vi "Write.vi"(7 "Wait Until Done?":bool, 8 "error in (no error)":errorcluster, 9 "Sample Rate [Hz]":dbl=1000.0 min=1000.0 max=1600000.0, 10 "Values":dbl[][](array[numeric]), 11 "AO (N Samples) Ref In":T1) -> (0 "error out":errorcluster, 3 "AO (N Samples) Ref Out":T1)   [LabVIEW 2021, in "AO Block.lvlib"]
doc: "Writes values to one or more analog output channels. Use this VI to write multiple samples for each channel at one time."
uses:
  <vilib>/myRIO/Instrument Drivers/Onboard IO/AO Block/AO Block.lvlib
  <vilib>/myRIO/Instrument Drivers/Onboard IO/AO Block/typedefs/AO Block Reference.ctl
  <vilib>/myRIO/Common/Instrument Driver Framework/Utilities/typedefs/myRIO Generic Hardware Reference.ctl
  <vilib>/myRIO/Common/Instrument Driver Framework/Utilities/typedefs/Hardware Version Enum.ctl
  <vilib>/myRIO/Common/Instrument Driver Framework/Utilities/typedefs/myRIO v1.0 Reference.ctl
  <vilib>/myRIO/Common/Instrument Driver Framework/Utilities/typedefs/Generic FPGA Reference.ctl
  <vilib>/myRIO/Common/Instrument Driver Framework/myRIO v1.0/AO Block/typedefs/AO Block Channels List.ctl
  <vilib>/myRIO/Common/Instrument Driver Framework/myRIO v1.0/AO Block/typedefs/AO Block Channels Enum.ctl
  <vilib>/myRIO/Common/Instrument Driver Framework/Utilities/typedefs/Analog Scaling Constants.ctl
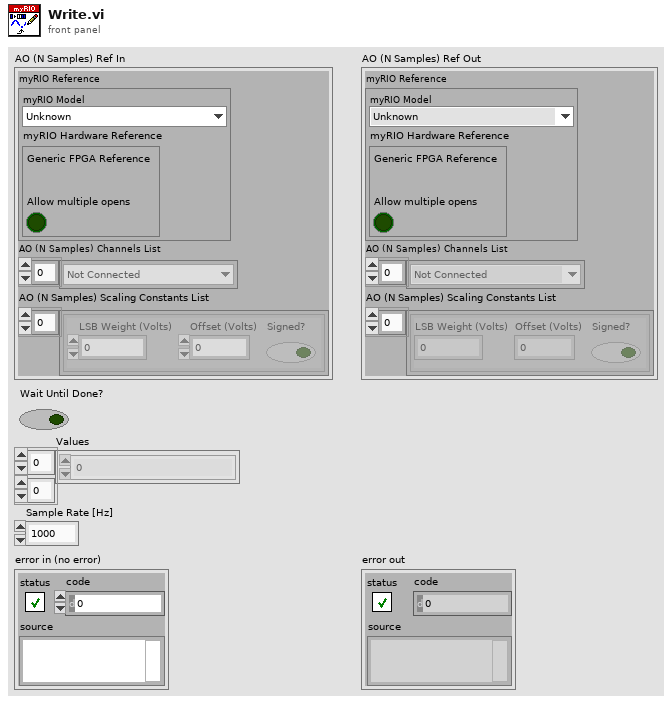
[diagram p1: front panel]
types:
  T1 = typedef "AO Block.lvlib/AO Block Reference.ctl" = cluster{"myRIO Reference":T2, "AO (N Samples) Channels List":T6, "AO (N Samples) Scaling Constants List":T8[]}
  T2 = typedef "myRIO Generic Hardware Reference.ctl" = cluster{"myRIO Model":T3, "myRIO Hardware Reference":T4}
  T3 = typedef "Hardware Version Enum.ctl" = enum16{"Unknown", "myRIO-1900", "myRIO-1950", "roboRIO", "NI ELVIS RIO CM", "ELVIS III"}
  T4 = typedef "myRIO v1.0 Reference.ctl" = cluster{"Generic FPGA Reference":T5, "Allow multiple opens":bool}
  T5 = typedef "Generic FPGA Reference.ctl" = refnum<k20>
  T6 = typedef "AO Block Channels List.ctl" = T7[]
  T7 = typedef "AO Block Channels Enum.ctl" = enum16{"Not Connected", "A/AO0 (N Samples)", "A/AO1 (N Samples)", "B/AO0 (N Samples)", "B/AO1 (N Samples)"}
  T8 = typedef "Analog Scaling Constants.ctl" = cluster{"LSB Weight (Volts)":dbl, "Offset (Volts)":dbl, "Signed?":bool}
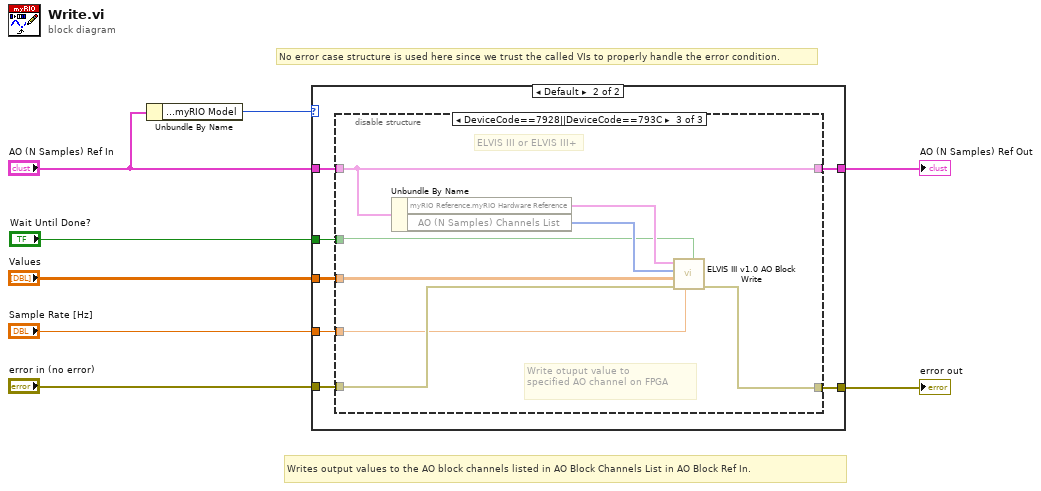
[diagram p0: block diagram]
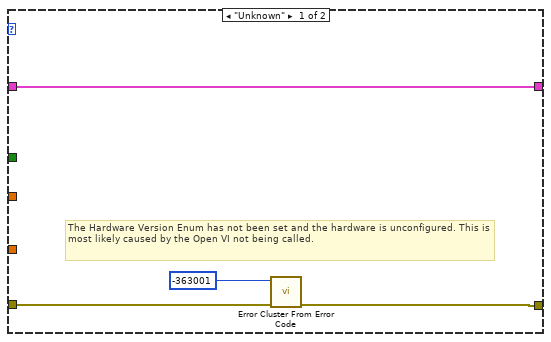
[diagram p2: hidden frame]
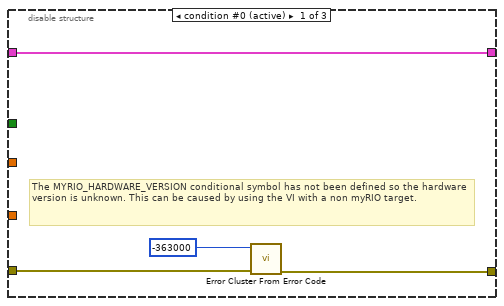
[diagram p3: hidden frame]
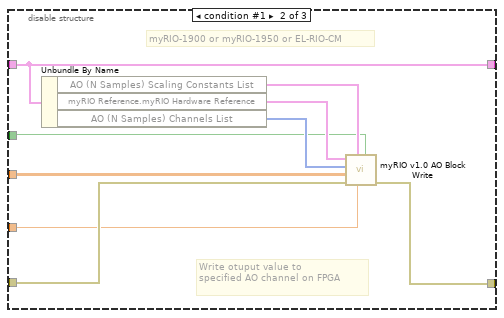
[diagram p4: hidden frame]
diagram:
  # "No error case structure is used here since we trust the called VIs to properly handle the error condition."
  # "Writes output values to the AO block channels listed in AO Block Channels List in AO Block Ref In."
  n1 = Unbundle By Name("AO (N Samples) Ref In") -> ("myRIO Reference.myRIO Model"=w3:T3)
  n2 = case shown="Default" w3 {
    tunnel: [w11 w19] -> w5
    tunnel: "AO (N Samples) Ref In" -> [w9 w18]
    tunnel: "error in (no error)" -> [w10 w17]
    tunnel: [w9 w16] -> w6
    tunnel: "Values" -> [_ w15]
    tunnel: "Sample Rate [Hz]" -> [_ w14]
    tunnel: "Wait Until Done?" -> [_ w13]
    frame "Unknown" {
      # "The Hardware Version Enum has not been set and the hardware is unconfigured. This is most likely caused by the Open VI not being called."
      n3 = call <vilib>:"Error Cluster From Error Code.vi"("error in (no error)"=w10, "error code (0)"=-363001) -> ("error out"=w11:errorcluster)  [unwired: 7 in]
    }
    frame Default {
      n4 = disable-structure shown="DeviceCode==7928||DeviceCode==793C" {
        disable-tunnel: w18 -> [w20 w26 w38]
        disable-tunnel: [w23 w30 w37] -> w19
        disable-tunnel: w17 -> [w21 w32 w36]
        disable-tunnel: [w20 w26 w38] -> w16
        disable-tunnel: w15 -> [_ w29 w34]
        disable-tunnel: w14 -> [_ w27 w35]
        disable-tunnel: w13 -> [_ w24 w33]
        frame condition #0 (active) {
          # "The MYRIO_HARDWARE_VERSION conditional symbol has not been defined so the hardware version is unknown. This can be caused by using the VI with a non myRIO target."
          n5 = call <vilib>:"Error Cluster From Error Code.vi"("error in (no error)"=w21, "error code (0)"=-363000) -> ("error out"=w23:errorcluster)  [unwired: 7 in]
        }
        frame condition #1 {
          # "myRIO-1900 or myRIO-1950 or EL-RIO-CM"
          # "Write otuput value to \nspecified AO channel on FPGA"
          n6 = Unbundle By Name(w26) -> ("AO (N Samples) Scaling Constants List"=w25:T8[], "myRIO Reference.myRIO Hardware Reference"=w28:T4, "AO (N Samples) Channels List"=w31:T6)
          n7 = call <vilib>:"myRIO v1.0 AO Block Write.vi"("Wait Until Done?"=w24, "AO FIFO Sample Rate"=w27, "Scale Constants Array"=w25, "error in (no error)"=w32, "dbl Scaled Value List"=w29, "AO (N Samples) Channel List"=w31, "myRIO Ref In"=w28) -> ("error out"=w30:errorcluster)  [unwired: 3 in, 1 out]
        }
        frame condition #2 {
          # "ELVIS III or ELVIS III+"
          # "Write otuput value to \nspecified AO channel on FPGA"
          n8 = Unbundle By Name(w38) -> ("myRIO Reference.myRIO Hardware Reference"=w39:T4, "AO (N Samples) Channels List"=w40:T6)
          n9 = call <vilib>:"ELVIS III v1.0 AO Block Write.vi"("Wait Until Done?"=w33, "AO FIFO Sample Rate"=w35, "error in (no error)"=w36, "dbl Scaled Value List"=w34, "AO (N Samples) Channel List"=w40, "myRIO Ref In"=w39) -> ("error out"=w37:errorcluster)  [unwired: 4 in, 1 out]
        }
      }
    }
  }
  "AO (N Samples) Ref Out" <- w6
  "error out" <- w5
